vi "Main - Footer eFGV.vi"(7 "Action":T1, 8 "error in":errorcluster, 11 "Footer in":string) -> (0 "error out":errorcluster, 2 "Footer Ref":refnum<user-event>, 3 "Footer out":string)   [LabVIEW 2019]
uses:
  Controls/eFGV States.ctl
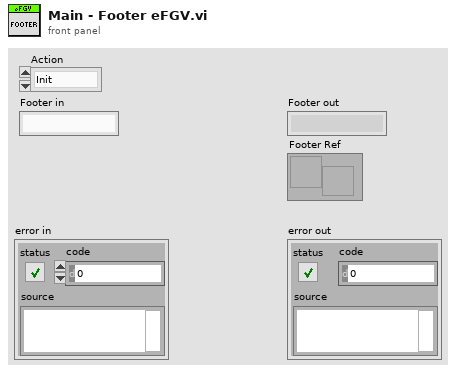
[diagram p1: front panel]
types:
  T1 = typedef "eFGV States.ctl" = enum16{"Init", "Read", "Write", "Exit"}
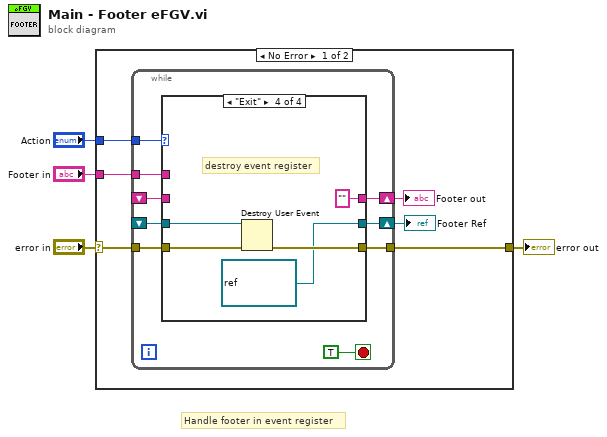
[diagram p0: block diagram]
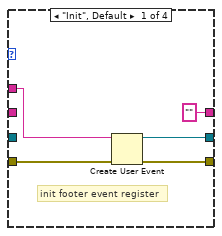
[diagram p2: hidden frame]
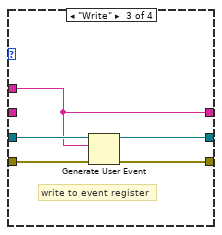
[diagram p4: hidden frame]
diagram:
  # "Handle footer in event register"
  n1 = case shown="No Error" "error in" {
    selector: "error in" -> [w7 w38]
    tunnel: "Action" -> [w10 _]
    tunnel: "Footer in" -> [w6 _]
    tunnel: [w9 w38] -> w2
    frame No Error {
      n2 = while {
        tunnel: w10 -> [w18]
        tunnel: w7 -> [w16]
        tunnel: [w15] -> w9
        shift-right: [w14] -> w8
        shift-left: _ -> [w13]
        shift-right: [w12] -> w5
        shift-left: _ -> [w17]
        tunnel: w6 -> [w11]
        stop <- TRUE stop-if-true
        n3 = case shown="\"Exit\"" w18 {
          tunnel: w17 -> [_ w25 _ _]
          tunnel: w16 -> [w24 w26 w32 w37]
          tunnel: [w23 w26 w31 w35] -> w15
          tunnel: [w22 w27 w29 refnum<user-event> refnum ("Footer in")] -> w14
          tunnel: w13 -> [_ w27 w30 w36]
          tunnel: ["" ("Footer in") w25 w28 "" ("Footer in")] -> w12
          tunnel: w11 -> [w21 _ w28 _]
          frame "Init", Default {
            # "init footer event register"
            n4 = Create User Event(user event datatype=w21, error in=w24) -> (user event=w22:refnum<user-event>, error out=w23:errorcluster)
          }
          frame "Read" {
            # "read from event register"
          }
          frame "Write" {
            # "write to event register"
            n5 = Generate User Event(user event=w30, event data cluster=w28, error in=w32) -> (user event out=w29:refnum<user-event>, error out=w31:errorcluster)  [unwired: 1 in]
          }
          frame "Exit" {
            # "destroy event register"
            n6 = Destroy User Event(user event=w36, error in=w37) -> (error out=w35:errorcluster)
          }
        }
      }
      "Footer Ref" <- w8
      "Footer out" <- w5
    }
    frame Error {
    }
  }
  "error out" <- w2
